vi "FTW-Connector-SpawnNewActor.vi"(0 "FTW Actor Connector Type":refnum<class "FTW-ActorConnector.lvclass">, 5 "Configuration":T2="{\n  \"Identity\": \"ActorName\",\n  \"InboxAddress\": \"tcp://127.0.0.1:*\",\n  \"PublisherAddress\": \"tcp://127.0.0.1:*\",\n  \"EnableInboxLogging\": true,\n  \"EnableJobLogging\": true,\n  \"DebugShowPanel\": false\n}", 7 "Actor VI Filepath":path, 9 "Timeout":i32=1000 format="%dmsec", 11 "error in":errorcluster) -> (4 "FTW Actor Connector":refnum<class "FTW-ActorConnector.lvclass">, 6 "Initialized Response":string, 8 "Instance Inbox Address":T1, 10 "Instance Publisher Address":T1, 15 "error out":errorcluster)   [LabVIEW 2012, in "FTW-Actor.lvlib" / "FTW-ActorConnector.lvclass"]
uses:
  FTW-ActorConnector.lvclass
  Utility/FTW-Actor-Configuration.ctl
  Utility/FTW-Actor-Address.ctl
  Endpoint/FTW-Endpoint.lvclass
  Core/JSON/FTW-JSON-RegexParse.vi
  Core/JSON/FTW-JSON-Format-Pair.vi
  Core/JSON/FTW-JSON-Format-String.vi
  Core/Regex/FTW-Regex.vi
  Core/JSON/FTW-JSON-RegexHeader.vi
  Core/Error/FTW-ERR-ThrowError.vi
  Core/JSON/FTW-JSON-Escape.vi
  Ether/FTW-Ether.lvclass
  FTW-Actor.lvlib
panel:
  # "Inputs"
  # "Outputs"
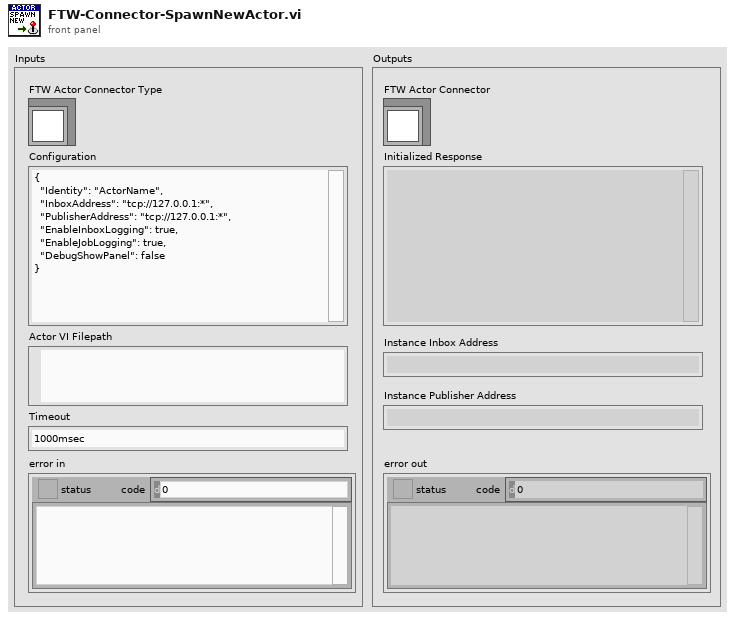
[diagram p1: front panel]
types:
  T1 = typedef "FTW-Actor.lvlib/FTW-Actor-Address.ctl" = string
  T2 = typedef "FTW-Actor.lvlib/FTW-Actor-Configuration.ctl" = string
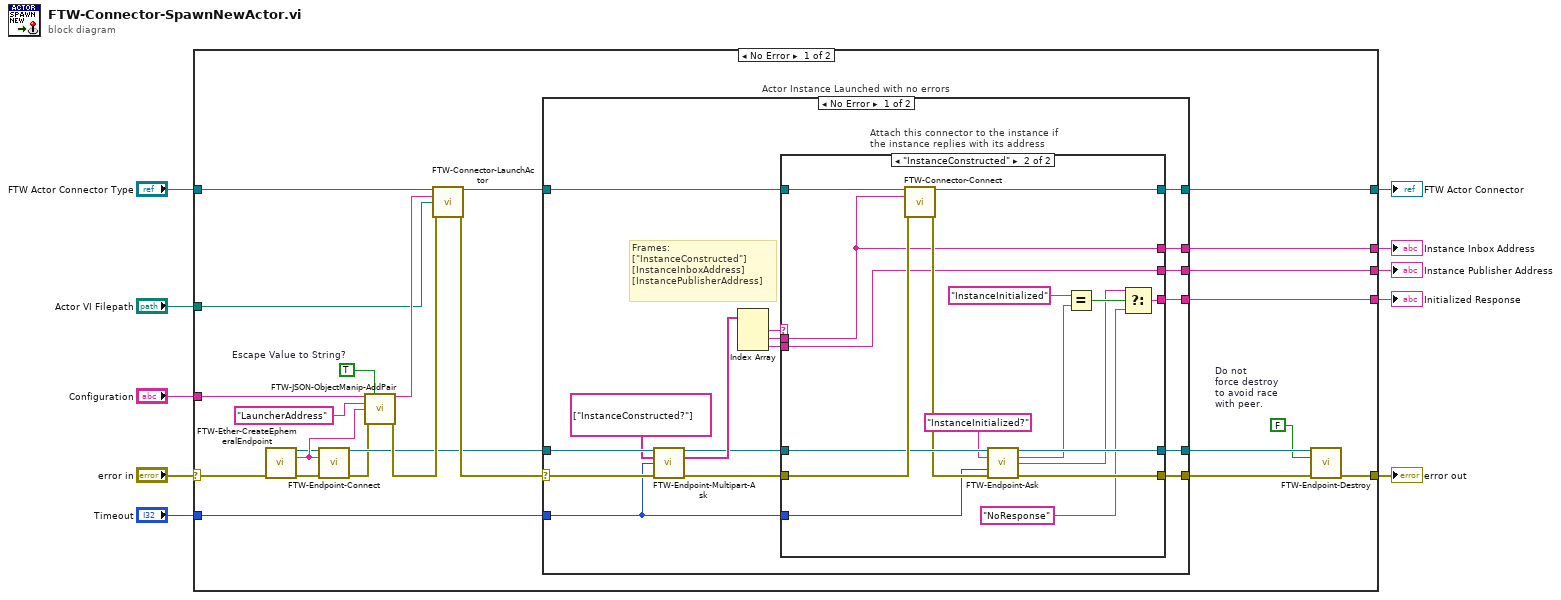
[diagram p0: block diagram]
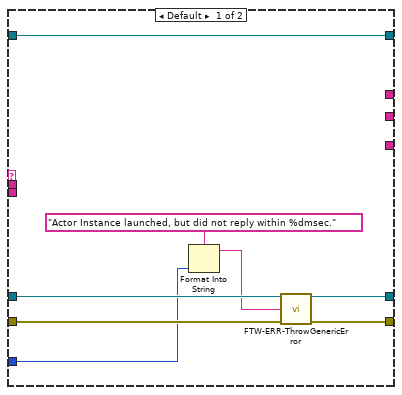
[diagram p2: hidden frame]
diagram:
  n1 = case shown="No Error" "error in" {
    selector: "error in" -> [w31 w80]
    tunnel: [w27 w80] -> w5
    tunnel: [w34 w79] -> w6
    tunnel: "FTW Actor Connector Type" -> [w24 w79]
    tunnel: "Configuration" -> [w33 _]
    tunnel: "Timeout" -> [w30 _]
    tunnel: "Actor VI Filepath" -> [w19 _]
    tunnel: [w18 _] -> w3
    tunnel: [w17 _] -> w2
    tunnel: [w16 _] -> w1
    frame No Error {
      w25 = FALSE  # Do not force destroy to avoid race with peer.
      w26 = TRUE  # Escape Value to String?
      n2 = call "FTW-Ether-CreateEphemeralEndpoint.vi"("error in"=w31) -> ("Ephemeral Endpoint"=w14:refnum<class "FTW-Endpoint.lvclass">, "Actual Ephemeral Address"=w15:T1, "error out"=w11:errorcluster)  [unwired: 12 in]
      n3 = call-dynamic "FTW-Endpoint-Connect.vi"("FTW Endpoint"=w14, "Endpoint Address"=w15, "error in"=w11) -> ("FTW Endpoint out"=w13:refnum<class "FTW-Endpoint.lvclass">, "error out"=w12:errorcluster)  [unwired: 11 in]
      n4 = call "FTW-JSON-ObjectManip-AddPair.vi"("Input JSON Object"=w33, "Escape Value to String?"=w26, "Key"="LauncherAddress", "Value"=w15, "error in"=w12) -> ("Output JSON Object"=w20:string, "error out"=w22:errorcluster)  [unwired: 9 in]
      n5 = call-dynamic "FTW-Connector-LaunchActor.vi"("FTW Actor Connector Type"=w24, "Configuration"=w20, "Actor VI Filepath"=w19, "error in"=w22) -> ("FTW Actor Connector"=w23:refnum<class "FTW-ActorConnector.lvclass">, "error out"=w21:errorcluster)  [unwired: 10 in]
      n6 = case "Actor Instance Launched with no errors" shown="No Error" w21 {
        selector: w21 -> [w43 w77]
        tunnel: [w51 w77] -> w28
        tunnel: w23 -> [w50 w78]
        tunnel: [w49 w78] -> w34
        tunnel: w13 -> [w44 w76]
        tunnel: w30 -> [w42 _]
        tunnel: [w48 w76] -> w29
        tunnel: [w37 _] -> w18
        tunnel: [w36 _] -> w17
        tunnel: [w35 _] -> w16
        frame No Error {
          # "Frames:\n[\"InstanceConstructed\"]\n[InstanceInboxAddress]\n[InstancePublisherAddress]"
          n7 = call-dynamic "FTW-Endpoint-Multipart-Ask.vi"("FTW Endpoint"=w44, "Multipart Message"=string[] ["InstanceConstructed?"], "Read Timeout"=w42, "error in"=w43) -> ("FTW Endpoint out"=w38:refnum<class "FTW-Endpoint.lvclass">, "Reply"=w40:string[], "error out"=w39:errorcluster)  [unwired: 7 in, 2 out]
          n8 = Index Array(array=w40) -> (element #1=w47:string, element #2=w46:string, element #3=w45:string)  [unwired: 3 in]
          n9 = case "Attach this connector to the instance if\nthe instance replies with its address" shown="\"InstanceConstructed\"" w47 {
            tunnel: [w56 w69] -> w51
            tunnel: w50 -> [w58 w74]
            tunnel: [w58 w73] -> w49
            tunnel: w38 -> [w55 w72]
            tunnel: w39 -> [w57 w75]
            tunnel: [w55 w71] -> w48
            tunnel: w42 -> [w53 w61]
            tunnel: w46 -> [_ w59]
            tunnel: w45 -> [_ w60]
            tunnel: [_ w62] -> w37
            tunnel: [_ w60] -> w36
            tunnel: [_ w59] -> w35
            frame Default {
              n10 = Format Into String(format string="Actor Instance launched, but did not reply within %dmsec." ("Error Message"), w53) -> (resulting string=w52:string)  [unwired: 2 in, 1 out]
              n11 = call "FTW-ERR-ThrowGenericError.vi"("Error Message"=w52, "error in"=w57) -> ("error out"=w56:errorcluster)  [unwired: 13 in]
            }
            frame "InstanceConstructed" {
              n12 = call-dynamic "FTW-Connector-Connect.vi"("FTW Actor Connector Type"=w74, "Instance Inbox Address"=w59, "error in"=w75) -> ("FTW Actor Connector"=w73:refnum<class "FTW-ActorConnector.lvclass">, "error out"=w70:errorcluster)  [unwired: 11 in]
              n13 = call-dynamic "FTW-Endpoint-Ask.vi"("FTW Endpoint"=w72, "Request Header"="InstanceInitialized?", "Timeout"=w61, "error in"=w70) -> ("FTW Endpoint out"=w71:refnum<class "FTW-Endpoint.lvclass">, "Response Header"=w66:string, "Response Body"=w64:string, "error out"=w69:errorcluster)  [unwired: 7 in, 1 out]
              n14 = Equal?(x="InstanceInitialized", y=w66) -> (x = y?=w65:bool)
              n15 = Select(t=w64, s=w65, f="NoResponse") -> (s? t:f=w62:string)
            }
          }
        }
        frame Error {
        }
      }
      n16 = call-dynamic "FTW-Endpoint-Destroy.vi"("FTW Endpoint"=w29, "Force Destroy"=w25, "error in"=w28) -> ("error out"=w27:errorcluster)  [unwired: 12 in]
    }
    frame Error {
    }
  }
  "error out" <- w5
  "FTW Actor Connector" <- w6
  "Initialized Response" <- w3
  "Instance Inbox Address" <- w1
  "Instance Publisher Address" <- w2
